vi "Tosca-Setup Devices.vi"(0 "Configuration file":path=path "C:/ProgramData/EPL/Tosca Defaults.ini", 2 "Parent VI":refnum<vi>, 7 "frame trigger?":bool) -> (6 "Changed":bool)   [LabVIEW 2020]
uses:
  TTL VIs/Typedefs/TTLControlledDevice XControl/TTLControlledDevice.xctl
  TTL VIs/Device Classes/Base Class/TTLControlledDevice.lvclass
  TTL VIs/Device Classes/WaterDelivery Class/TTLWaterDelivery.lvclass
  epl-vi-lib/Utility VIs/Controls/KTable/KTable.xctl
  TTL VIs/Device Classes/Base Class/TTLControlledDevice.lvclass/TTLControlledDevice.ctl
  epl-vi-lib/Connection VIs/Typedefs/CM-Endpoint.ctl
  e799b8b4-95e5-4a75-bcd5-f4c261b377d9.vi
  5e81ef1a-d4e7-4bbe-bc92-e5df060631d5.vi
  TTL VIs/Device Classes/Base Class/Read Name.vi
  TTL VIs/Device Classes/Base Class/Write Name.vi
  epl-vi-lib/Utility VIs/File IO VIs/Configuration File Wrapper VIs/Config-Read Key (string).vi
  epl-vi-lib/Utility VIs/File IO VIs/Configuration File Wrapper VIs/Config-Write Key (string).vi
  <vilib>/Comparison/Equal/Equal Functor/Equal Functor.lvclass
panel:
  in  "Add Button":bool
  in  "DO Port":u16(ring)=7 caption="Digital Output Port" items=["PXI1Slot3/port0"]
  in  "DI Port":u16(ring)=6 caption="Digital Input Port" items=["PXI1Slot3/port0", "PXI1Slot3/port1", "PXI1Slot3/port2"]
  in  "DO":u16(xcontrol)
  in  "DI":u16(xcontrol)
  in  "AO":u16(xcontrol)
  in  "AI":u16(xcontrol)
  in  "Apply Button":bool
  in  "Exit":bool
  in  "DigDevice 2":refnum<class "TTLControlledDevice.lvclass">(xcontrol)
  in  "DigDevice 1":refnum<class "TTLControlledDevice.lvclass">(xcontrol)=refnum
  in  "DigDevice 0":refnum<class "TTLControlledDevice.lvclass">(xcontrol)=refnum
  # "ANALOG"
  # "TTL-Controlled Devices"
  # "DIGITAL"
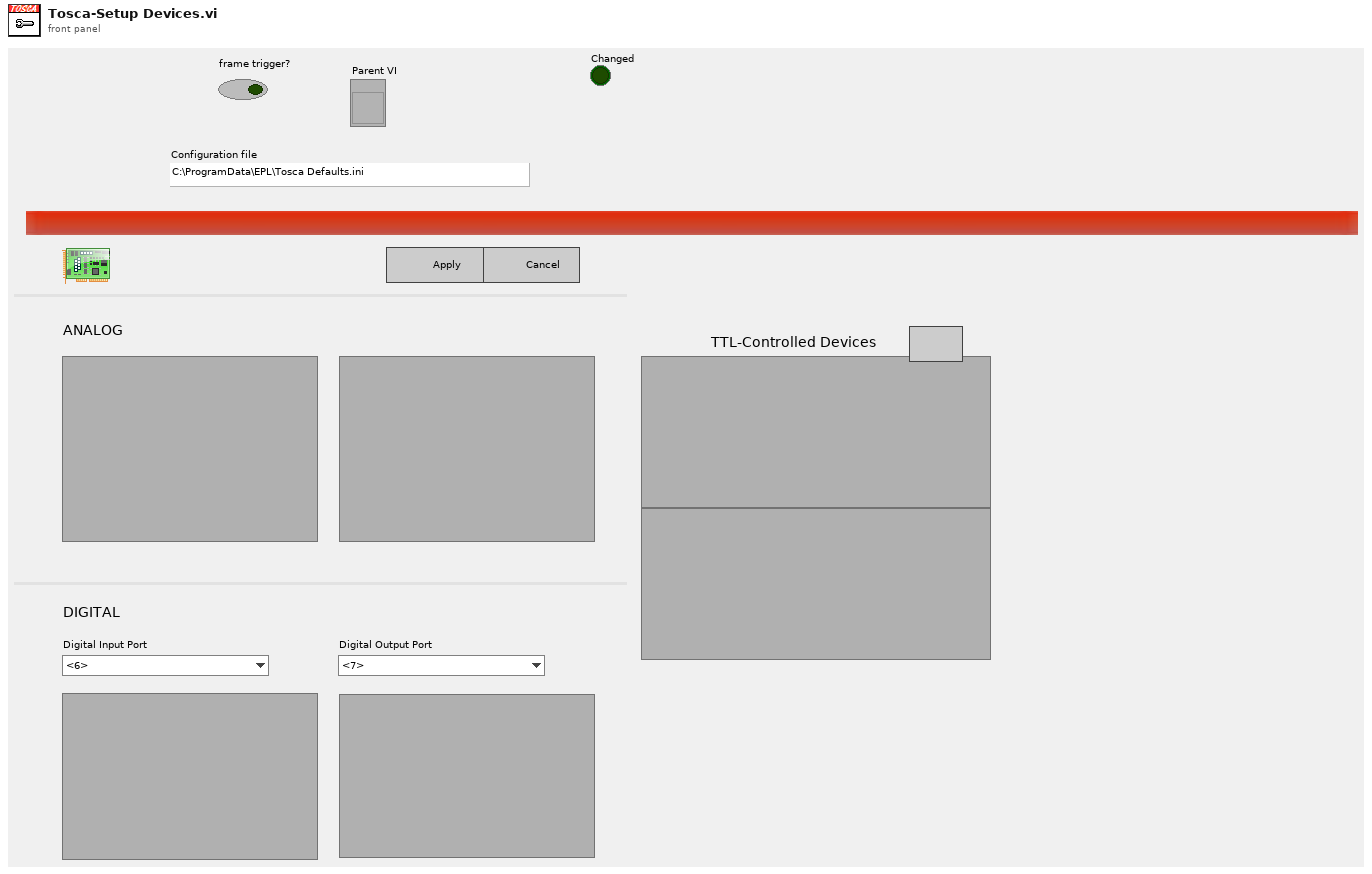
[diagram p1: front panel]
types:
  T1 = enum16{"Left Button", "Center Button", "Right Button", "Window Close"}
  T2 = typedef "CM-Endpoint.ctl" = cluster{"Name":string, "Device":string}
  T3 = enum8{"Enabled", "Disabled", "Disabled and Grayed Out"}
  T4 = typedef "CM-Connection.ctl" = cluster{"IOChannel":string, "Endpoint":string}
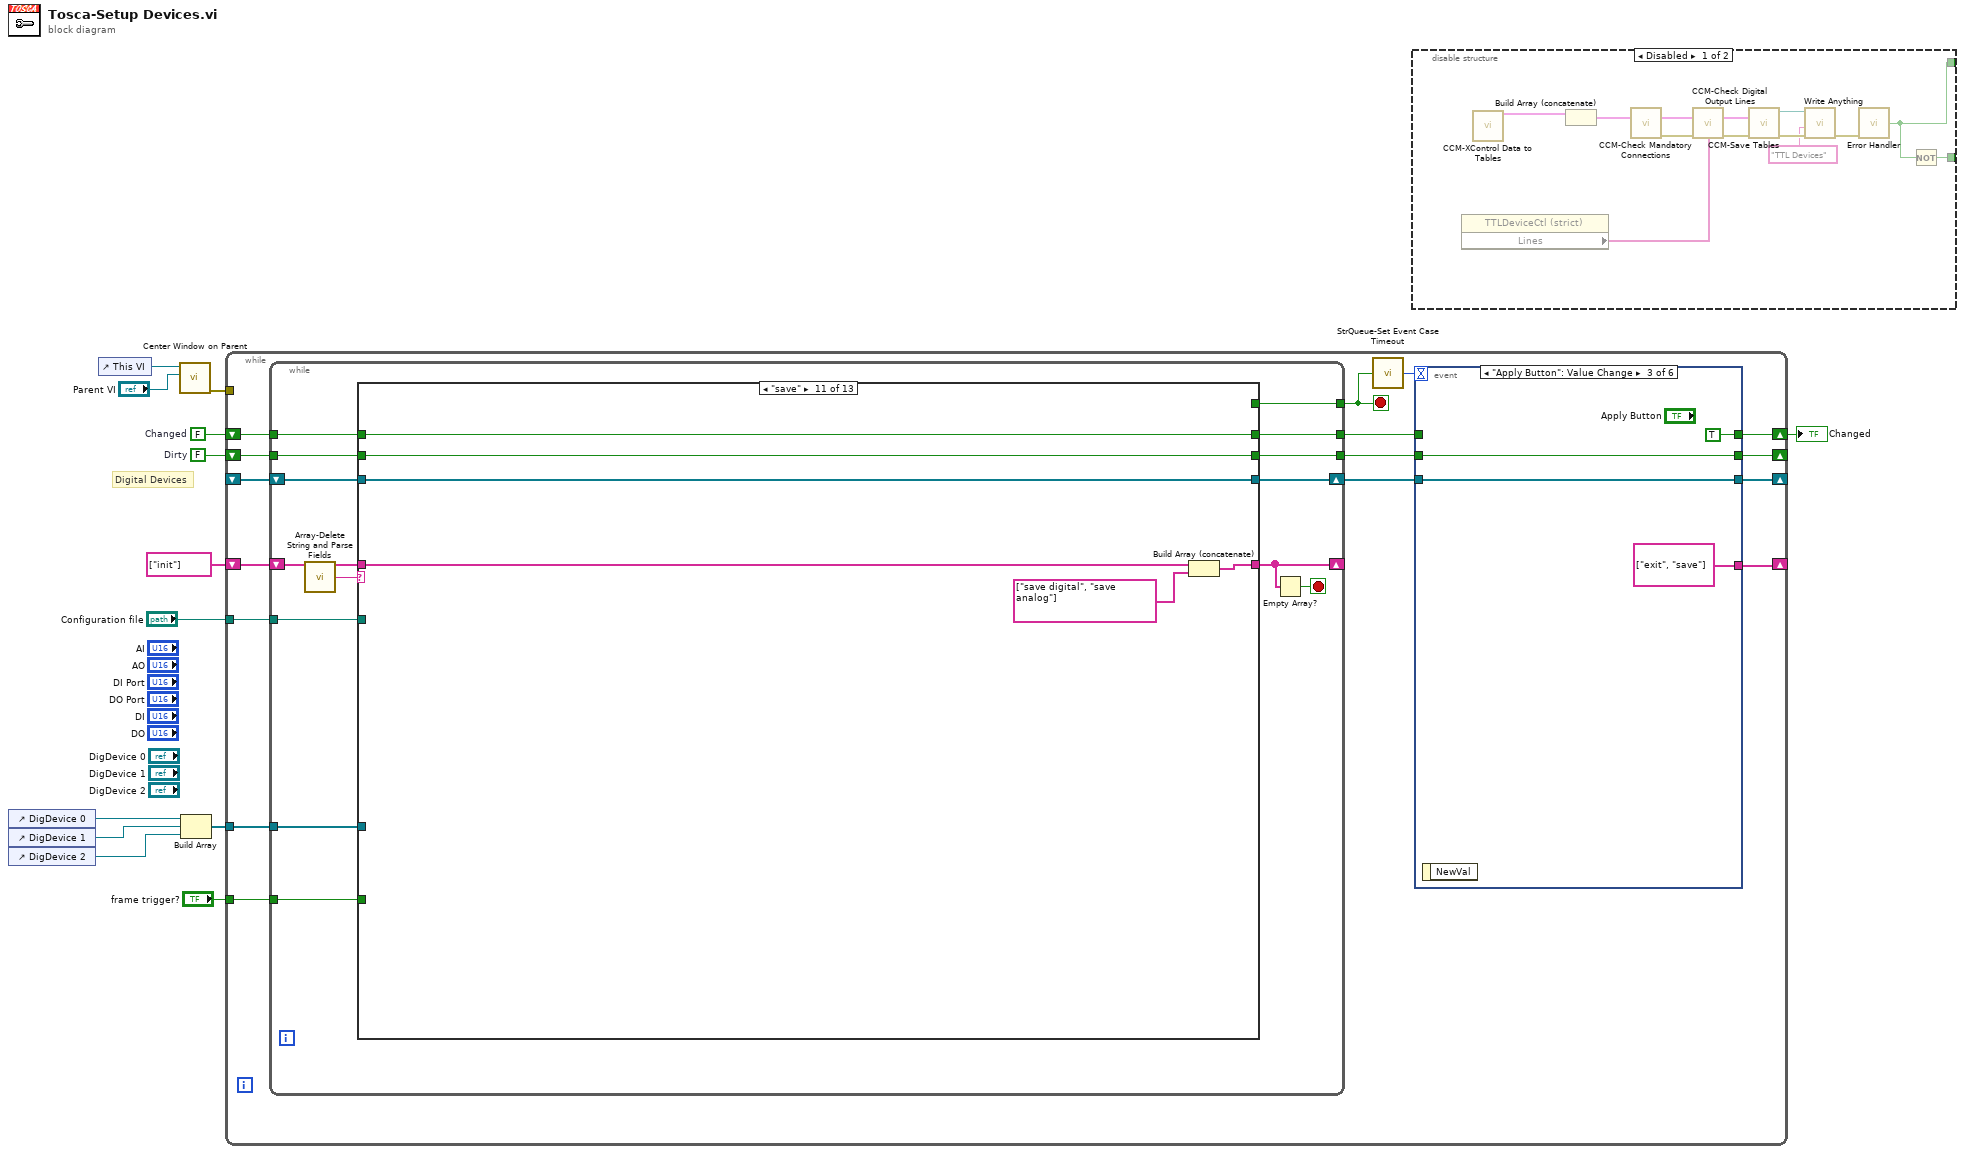
[diagram p0: block diagram]
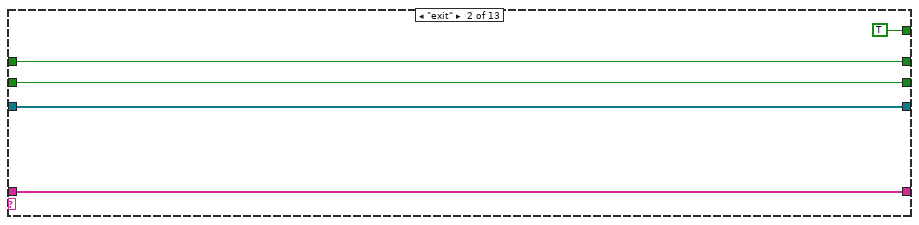
[diagram p3: hidden frame]
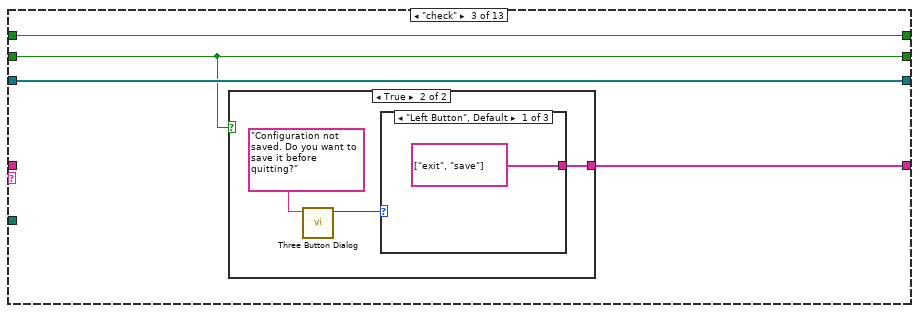
[diagram p4: hidden frame]
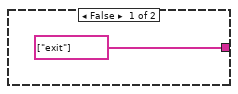
[diagram p5: hidden frame]
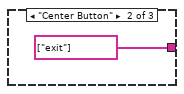
[diagram p6: hidden frame]
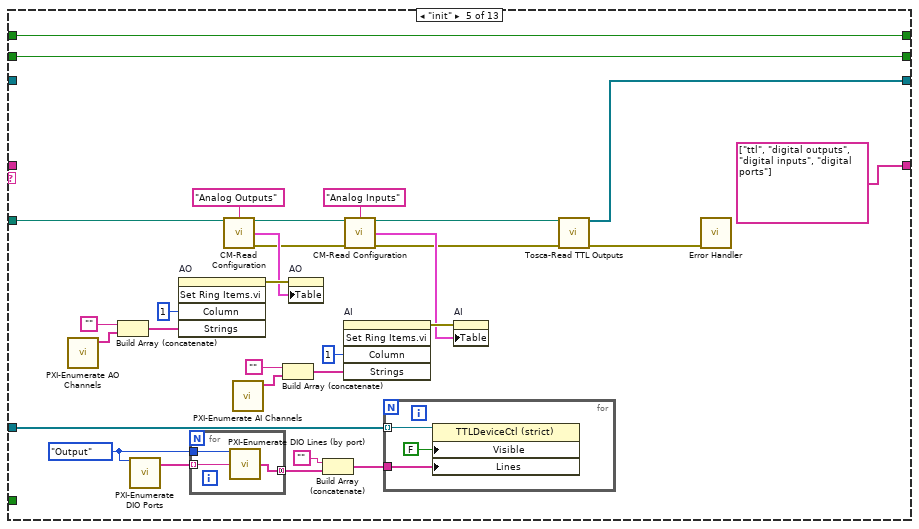
[diagram p9: hidden frame]
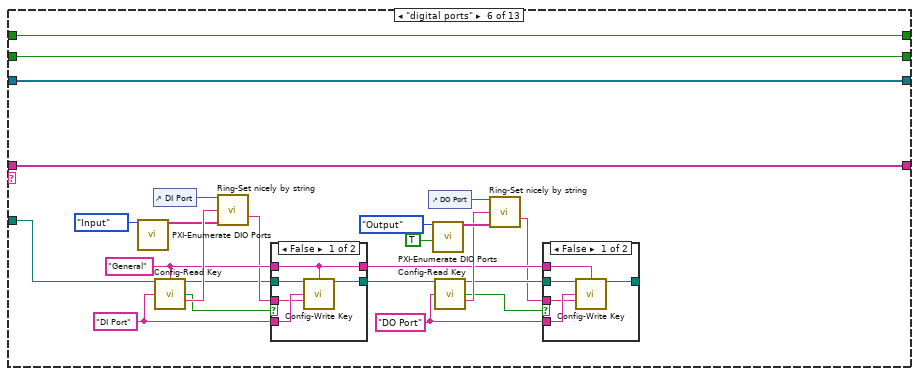
[diagram p10: hidden frame]
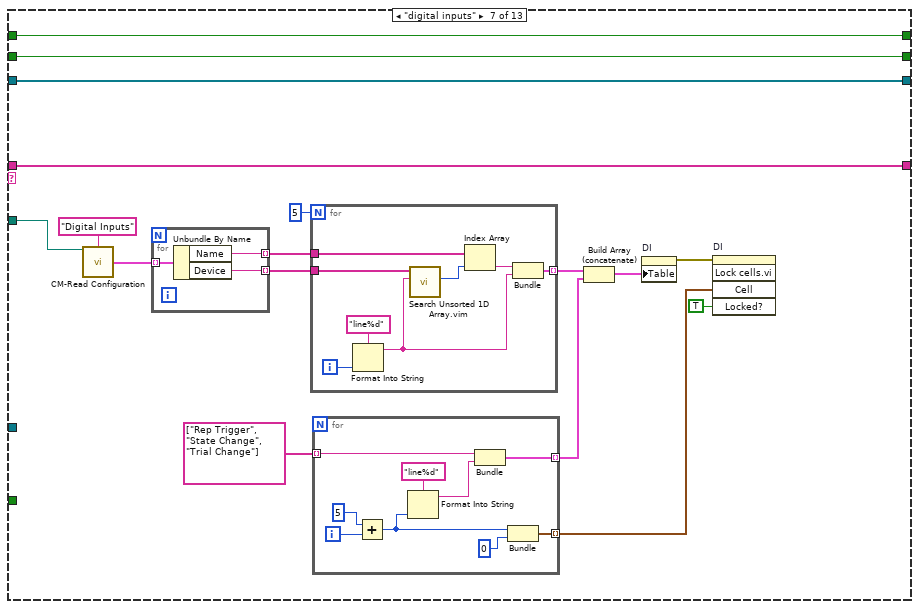
[diagram p13: hidden frame]
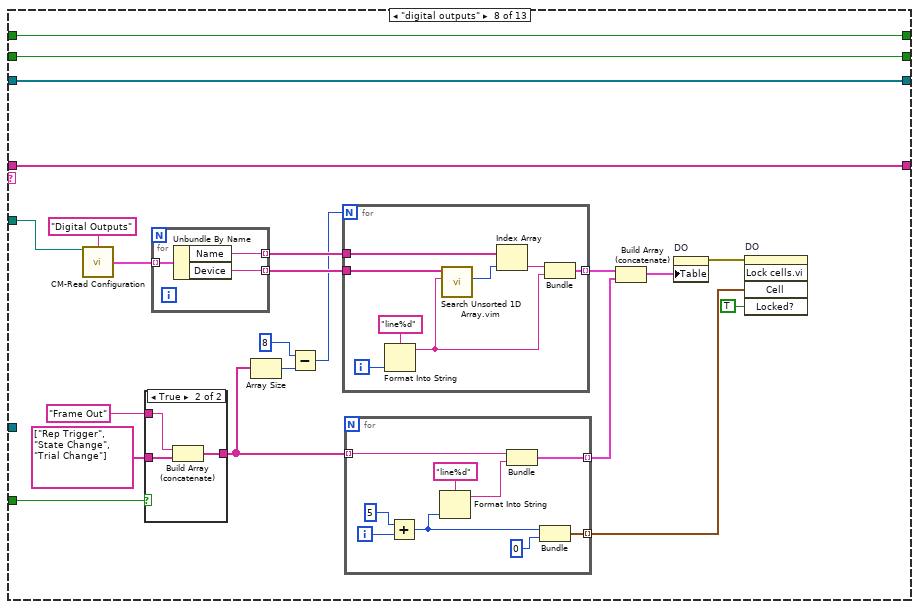
[diagram p14: hidden frame]
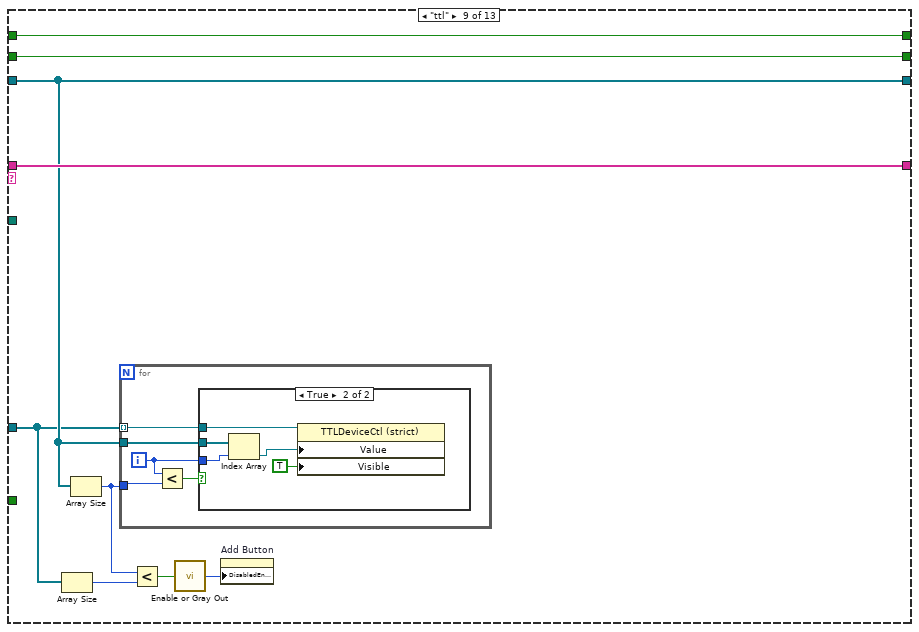
[diagram p16: hidden frame]
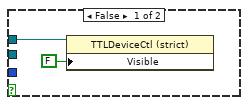
[diagram p17: hidden frame]
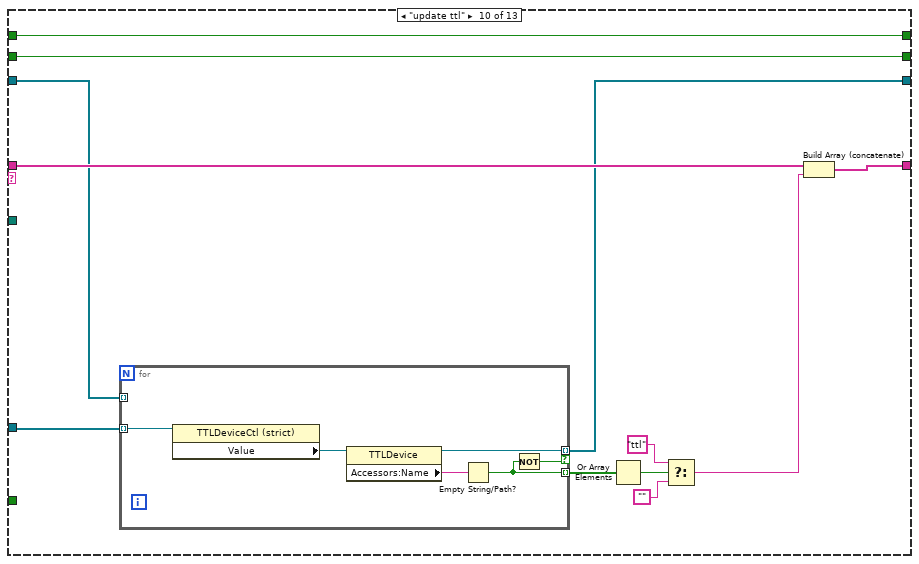
[diagram p18: hidden frame]
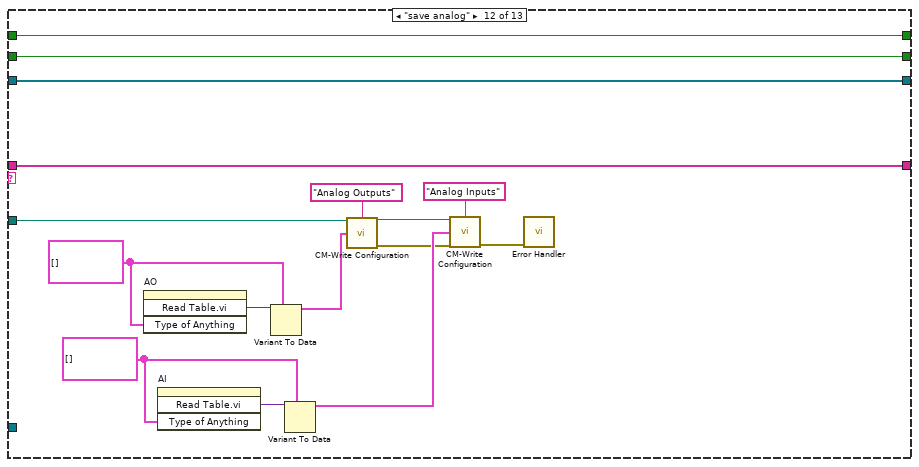
[diagram p19: hidden frame]
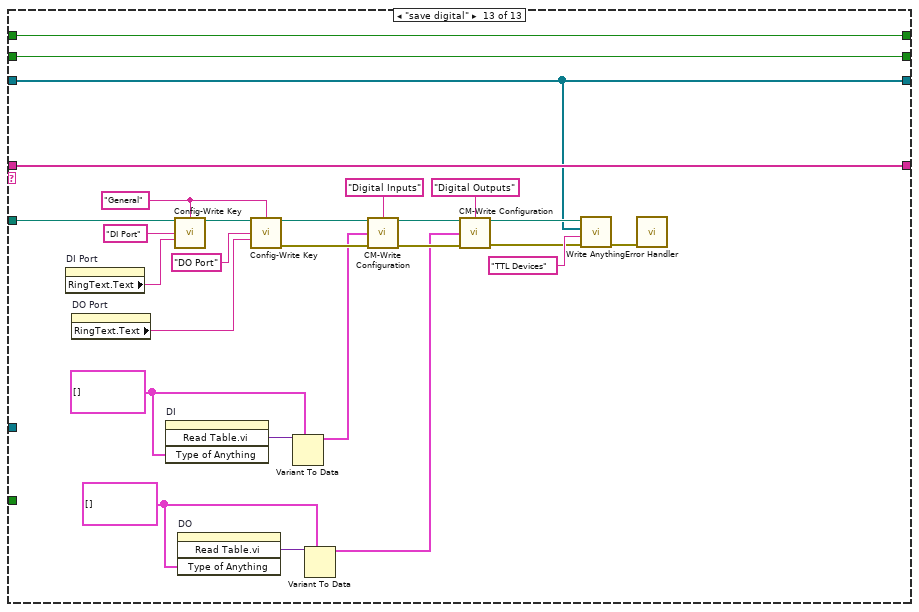
[diagram p20: hidden frame]
diagram:
  w11 = FALSE  # Changed
  w12 = FALSE  # Dirty
  # "Digital Devices"
  n1 = control-ref of="DigDevice 0"() -> (w9:refnum<vi>)
  n2 = control-ref of="DigDevice 1"() -> (w8:refnum<vi>)
  n3 = control-ref of="DigDevice 2"() -> (w7:refnum<vi>)
  n4 = control-ref of="This VI"() -> (w2:refnum<vi>)
  n5 = call "Center Window on Parent.vi"("Parent VI"="Parent VI", "VI in"=w2) -> ("error out"=w4:errorcluster)  [unwired: 8 in, 1 out]
  n6 = Build Array(w9, w8, w7) -> (w6:refnum<vi>[])
  n7 = while {
    shift-right: [w22] -> _
    shift-left: w12 -> [w27]
    tunnel: "Configuration file" -> [w16]
    shift-right: [w21] -> w10
    shift-left: w11 -> [w28]
    tunnel: w6 -> [w14]
    shift-right: [w23] -> _
    shift-left: _ -> [w26]
    shift-right: [w18] -> _
    shift-left: string[] ["init"] -> [w29]
    tunnel: w4 -> [_]
    tunnel: "frame trigger?" -> [w15]
    stop <- w24 stop-if-true
    n8 = while {
      shift-right: [w44] -> _
      shift-left: w29 -> [w41]
      tunnel: [w42] -> w24
      tunnel: w28 -> [w38]
      tunnel: w27 -> [w37]
      tunnel: [w35] -> w20
      tunnel: [w34] -> w19
      tunnel: w16 -> [w30]
      tunnel: w15 -> [w32]
      tunnel: w14 -> [w31]
      shift-right: [w33] -> w17
      shift-left: w26 -> [w36]
      stop <- w43 stop-if-true
      n9 = call "Array-Delete String and Parse Fields.vi"("Array in"=w41) -> ("Array out"=w40:string[], "Field 1"=w39:string)  [unwired: 10 in, 3 out]
      n10 = case shown="\"save\"" w39 {
        tunnel: w40 -> [w48 w53 _ w67 _ w105 w155 w197 w233 w257 w269 w285 w312]
        tunnel: [w48 w53 w54 w67 string[] ["ttl", "digital outputs", "digital inputs", "digital ports"] ("Array out") w105 w155 w197 w233 w251 w265 w285 w312] -> w44
        tunnel: [_ TRUE _ _ _ _ _ _ _ _ _ _ _] -> w42
        tunnel: w38 -> [w47 w51 w57 w66 w97 w128 w158 w200 w232 w256 w268 w284 w311]
        tunnel: w37 -> [w46 w50 w55 w65 w96 w127 w157 w199 w231 w255 w267 w283 w310]
        tunnel: w36 -> [w45 w49 w56 w64 _ w126 w156 w198 w230 w254 w266 w282 w289]
        tunnel: [w47 w51 w57 w66 w97 w128 w158 w200 w232 w256 w268 w284 w311] -> w35
        tunnel: [w46 w50 w55 w65 w96 w127 w157 w199 w231 w255 w267 w283 w310] -> w34
        tunnel: [w45 w49 w56 w64 w68 w126 w156 w198 w230 w252 w266 w282 w289] -> w33
        tunnel: w30 -> [_ _ _ _ w95 w104 w153 w195 _ _ _ w277 w307]
        tunnel: w32 -> [_ _ _ _ _ _ _ w184 _ _ _ _ _]
        tunnel: w31 -> [_ _ _ _ w72 _ _ _ w229 w253 _ _ _]
        frame "", Default {
        }
        frame "exit" {
        }
        frame "check" {
          n11 = case shown="True" w55 {
            tunnel: [string[] ["exit"] w59] -> w54
            frame False {
            }
            frame True {
              n12 = call <vilib>:"Three Button Dialog.vi"("message"="Configuration not saved. Do you want to save it before quitting?") -> ("Which Button?"=w60:T1)  [unwired: 10 in]
              n13 = case shown="\"Left Button\", Default" w60 {
                tunnel: [string[] ["exit", "save"] string[] ["exit"] _] -> w59
                frame "Left Button", Default {
                }
                frame "Center Button" {
                }
                frame "Right Button" {
                }
              }
            }
          }
        }
        frame "load" {
        }
        frame "init" {
          w75 = enum16{"Input", "Output"}."Output" ("Direction")
          n14 = call "PXI-Enumerate AO Channels.vi"() -> ("AO.PhysicalChans"=w92:tag[])  [unwired: 10 in, 1 out]
          n15 = Build Array (concatenate)("", w92) -> (w90:string[])
          n16 = call "PXI-Enumerate DIO Ports.vi"("Direction"=w75) -> ("Ports"=w74:tag[])  [unwired: 13 in, 1 out]
          n17 = invoke on="AO" class="KTable (strict)" method="Set Ring Items.vi"("Column"=1, "Strings"=w90) -> (error out=w94:errorcluster)  [unwired: 3 in, 4 out]
          n18 = for {
            tunnel: w74 -> [w99] mode=indexing
            tunnel: w75 -> [w100]
            tunnel: [w98] -> w76 mode=concatenating
            n19 = call "PXI-Enumerate DIO Lines (by port).vi"("Direction"=w100, "Port"=w99) -> ("Dev/Port/Lines"=w98:tag[])  [unwired: 11 in, 2 out]
          }
          n20 = call "CM-Read Configuration.vi"("Connection File Path"=w95, "Section"="Analog Outputs") -> ("Connection File Path thru"=w86:path, "Endpoints"=w89:T2[], "error out"=w85:errorcluster)  [unwired: 9 in, 2 out]
          n21 = call "PXI-Enumerate AI Channels.vi"() -> ("AI.PhysicalChans"=w82:tag[])  [unwired: 10 in, 1 out]
          n22 = Build Array (concatenate)("", w82) -> (w80:string[])
          n23 = property on="AO" class="KTable (strict)"(error in=w94, "Table"=w89) -> ()  [unwired: 1 in, 2 out]
          n24 = Build Array (concatenate)("", w76) -> (w77:string[])
          n25 = invoke on="AI" class="KTable (strict)" method="Set Ring Items.vi"("Column"=1, "Strings"=w80) -> (error out=w84:errorcluster)  [unwired: 3 in, 4 out]
          n26 = call "CM-Read Configuration.vi"("Connection File Path"=w86, "Section"="Analog Inputs", "error in (no error)"=w85) -> ("Connection File Path thru"=w71:path, "Endpoints"=w79:T2[], "error out"=w69:errorcluster)  [unwired: 8 in, 2 out]
          n27 = for {
            tunnel: w77 -> [w102]
            tunnel: w72 -> [w101] mode=indexing
            n28 = property class="TTLDeviceCtl (strict)"(reference=w101, "Visible"=FALSE, "Lines"=w102) -> ()  [unwired: 1 in, 2 out]
          }
          n29 = property on="AI" class="KTable (strict)"(error in=w84, "Table"=w79) -> ()  [unwired: 1 in, 2 out]
          n30 = call "Tosca-Read TTL Outputs.vi"("Connection File Path thru"=w71, "error in (no error)"=w69) -> ("Devices"=w68:refnum<class "TTLControlledDevice.lvclass">[], "error out"=w70:errorcluster)  [unwired: 12 in]
          n31 = call "Error Handler.vi"("error in (no error)"=w70) -> ()  [unwired: 12 in, 3 out]
        }
        frame "digital ports" {
          w110 = "DO Port" ("key")
          w116 = "DI Port" ("key")
          w117 = "General" ("section")
          n32 = call "PXI-Enumerate DIO Ports.vi"("Direction"=enum16{"Input", "Output"}."Input") -> ("Ports"=w121:tag[])  [unwired: 13 in, 1 out]
          n33 = control-ref of="DI Port"() -> (w107:refnum<vi>)
          n34 = call-poly "Config-Read Key.vi"("configuration file path"=w104, "section"=w117, "key"=w116) -> ("file path"=w114:path, "found?"=w118:bool, "value"=w122:string)  [unwired: 9 in, 1 out]
          n35 = call "Ring-Set nicely by string.vi"("Ring in"=w107, "Device"=w122, "Strings []"=w121) -> ("Selection"=w115:string)  [unwired: 8 in, 4 out]
          n36 = case shown="False" w118 {
            tunnel: w117 -> [w137 w141]
            tunnel: w116 -> [w139 _]
            tunnel: w115 -> [w138 _]
            tunnel: [w137 w141] -> w112
            tunnel: w114 -> [w136 w140]
            tunnel: [w135 w140] -> w113
            frame False {
              n37 = call-poly "Config-Write Key.vi"("configuration file path"=w136, "section"=w137, "key"=w139, "value"=w138) -> ("file path"=w135:path)  [unwired: 9 in, 2 out]
            }
            frame True {
            }
          }
          n38 = control-ref of="DO Port"() -> (w106:refnum<vi>)
          n39 = call "PXI-Enumerate DIO Ports.vi"("Direction"=enum16{"Input", "Output"}."Output", "Must be buffered"=TRUE) -> ("Ports"=w120:tag[])  [unwired: 12 in, 1 out]
          n40 = call-poly "Config-Read Key.vi"("configuration file path"=w113, "key"=w110) -> ("file path"=w111:path, "found?"=w108:bool, "value"=w119:string)  [unwired: 10 in, 1 out]
          n41 = call "Ring-Set nicely by string.vi"("Ring in"=w106, "Device"=w119, "Strings []"=w120) -> ("Selection"=w109:string)  [unwired: 8 in, 4 out]
          n42 = case shown="False" w108 {
            tunnel: w112 -> [w131 _]
            tunnel: w110 -> [w133 _]
            tunnel: w109 -> [w132 _]
            tunnel: w111 -> [w130 w134]
            tunnel: [w129 w134] -> _
            frame False {
              n43 = call-poly "Config-Write Key.vi"("configuration file path"=w130, "section"=w131, "key"=w133, "value"=w132) -> ("file path"=w129:path)  [unwired: 9 in, 2 out]
            }
            frame True {
            }
          }
        }
        frame "digital inputs" {
          n44 = call "CM-Read Configuration.vi"("Connection File Path"=w153, "Section"="Digital Inputs") -> ("Endpoints"=w152:T2[])  [unwired: 9 in, 4 out]
          n45 = for {
            tunnel: w152 -> [w178] mode=indexing
            tunnel: [w177] -> w150 mode=indexing
            tunnel: [w176] -> w149 mode=indexing
            n46 = Unbundle By Name(w178) -> ("Name"=w177:string, "Device"=w176:string)
          }
          n47 = for {
            N: 5 -> [_]
            tunnel: w150 -> [w172]
            tunnel: w149 -> [w173]
            tunnel: [w168] -> w147 mode=indexing
            i -> [w175]
            n48 = Format Into String(format string="line%d", w175) -> (resulting string=w169:string)  [unwired: 2 in, 1 out]
            n49 = call "Search Unsorted 1D Array.vim"("element"=w169, "unsorted 1D array"=w173) -> ("index of element"=w171:i32)  [unwired: 9 in]
            n50 = Index Array(array=w172, index=w171) -> (element=w170:string)
            n51 = Bundle("Name"=w170, w169) -> (w168:cluster{"Name":string, string})  [unwired: 1 in]
          }
          n52 = for {
            tunnel: string[] ["Rep Trigger", "State Change", "Trial Change"] -> [w163] mode=indexing
            tunnel: [w164] -> w146 mode=indexing
            tunnel: [w159] -> w143 mode=indexing
            i -> [w167]
            n53 = Add(x=5, y=w167) -> (x+y=w161:i32)
            n54 = Format Into String(format string="line%d", w161) -> (resulting string=w165:string)  [unwired: 2 in, 1 out]
            n55 = Bundle("String"=w163, w165) -> (w164:cluster{"String":string, string})  [unwired: 1 in]
            n56 = Bundle(w161, 0) -> (w159:cluster{i32, i32})  [unwired: 1 in]
          }
          n57 = Build Array (concatenate)(w147, w146) -> (w145:cluster{"String":string, string}[])
          n58 = property on="DI" class="KTable (strict)"("Table"=w145) -> (error out=w144:errorcluster)  [unwired: 2 in, 1 out]
          n59 = invoke on="DI" class="KTable (strict)" method="Lock cells.vi"(error in=w144, "Cell"=w143, "Locked?"=TRUE) -> ()  [unwired: 2 in, 5 out]
        }
        frame "digital outputs" {
          n60 = call "CM-Read Configuration.vi"("Connection File Path"=w195, "Section"="Digital Outputs") -> ("Endpoints"=w194:T2[])  [unwired: 9 in, 4 out]
          n61 = case shown="True" w184 {
            tunnel: string[] ["Rep Trigger", "State Change", "Trial Change"] -> [w201 w204]
            tunnel: [w201 w203] -> w181
            tunnel: "Frame Out" ("String") -> [_ w202]
            frame False {
            }
            frame True {
              n62 = Build Array (concatenate)(w202, w204) -> (w203:string[])
            }
          }
          n63 = for {
            tunnel: w194 -> [w224] mode=indexing
            tunnel: [w223] -> w193 mode=indexing
            tunnel: [w222] -> w192 mode=indexing
            n64 = Unbundle By Name(w224) -> ("Name"=w223:string, "Device"=w222:string)
          }
          n65 = Array Size(array=w181) -> (size(s)=w182:i32)
          n66 = Subtract(x=8, y=w182) -> (x-y=w179:i32)
          n67 = for {
            N: w179 -> [_]
            tunnel: w193 -> [w218]
            tunnel: w192 -> [w219]
            tunnel: [w214] -> w191 mode=indexing
            i -> [w221]
            n68 = Format Into String(format string="line%d", w221) -> (resulting string=w215:string)  [unwired: 2 in, 1 out]
            n69 = call "Search Unsorted 1D Array.vim"("element"=w215, "unsorted 1D array"=w219) -> ("index of element"=w217:i32)  [unwired: 9 in]
            n70 = Index Array(array=w218, index=w217) -> (element=w216:string)
            n71 = Bundle("Name"=w216, w215) -> (w214:cluster{"Name":string, string})  [unwired: 1 in]
          }
          n72 = for {
            tunnel: w181 -> [w209] mode=indexing
            tunnel: [w210] -> w190 mode=indexing
            tunnel: [w205] -> w187 mode=indexing
            i -> [w213]
            n73 = Add(x=5, y=w213) -> (x+y=w207:i32)
            n74 = Format Into String(format string="line%d", w207) -> (resulting string=w211:string)  [unwired: 2 in, 1 out]
            n75 = Bundle("String"=w209, w211) -> (w210:cluster{"String":string, string})  [unwired: 1 in]
            n76 = Bundle(w207, 0) -> (w205:cluster{i32, i32})  [unwired: 1 in]
          }
          n77 = Build Array (concatenate)(w191, w190) -> (w189:cluster{"String":string, string}[])
          n78 = property on="DO" class="KTable (strict)"("Table"=w189) -> (error out=w188:errorcluster)  [unwired: 2 in, 1 out]
          n79 = invoke on="DO" class="KTable (strict)" method="Lock cells.vi"(error in=w188, "Cell"=w187, "Locked?"=TRUE) -> ()  [unwired: 2 in, 5 out]
        }
        frame "ttl" {
          n80 = Array Size(array=w229) -> (size(s)=w227:i32)
          n81 = Array Size(array=w230) -> (size(s)=w228:i32)
          n82 = for {
            tunnel: w228 -> [w238]
            tunnel: w230 -> [w235]
            tunnel: w229 -> [w234] mode=indexing
            i -> [w236]
            n83 = Less?(x=w236, y=w238) -> (x < y?=w237:bool)
            n84 = case shown="True" w237 {
              tunnel: w236 -> [_ w245]
              tunnel: w235 -> [_ w243]
              tunnel: w234 -> [w239 w241]
              frame False {
                n85 = property class="TTLDeviceCtl (strict)"(reference=w239, "Visible"=FALSE) -> ()  [unwired: 1 in, 2 out]
              }
              frame True {
                n86 = Index Array(array=w243, index=w245) -> (element=w242:refnum<class "TTLControlledDevice.lvclass">)
                n87 = property class="TTLDeviceCtl (strict)"(reference=w241, "Value"=w242, "Visible"=TRUE) -> ()  [unwired: 1 in, 2 out]
              }
            }
          }
          n88 = Less?(x=w228, y=w227) -> (x < y?=w226:bool)
          n89 = call "Enable or Gray Out.vi"("Boolean"=w226) -> ("Disabled"=w225:T3)
          n90 = property on="Add Button" class="Bool"("DisabledEnum"=w225) -> ()  [unwired: 2 in, 2 out]
        }
        frame "update ttl" {
          n91 = for {
            tunnel: w254 -> [_] mode=indexing
            tunnel: w253 -> [w263] mode=indexing
            tunnel: [w260] -> w252 mode=indexing if=w259
            tunnel: [w258] -> w250 mode=indexing
            n92 = property class="TTLDeviceCtl (strict)"(reference=w263) -> ("Value"=w262:refnum<class "TTLControlledDevice.lvclass">)  [unwired: 1 in, 2 out]
            n93 = property class="TTLDevice"(reference=w262) -> (reference out=w260:refnum<class "TTLControlledDevice.lvclass">, "Accessors:Name"=w261:string)  [unwired: 1 in, 1 out]
            n94 = Empty String/Path?(string/path=w261) -> (empty?=w258:bool)
            n95 = Not(x=w258) -> (.not. x?=w259:bool)
          }
          n96 = Or Array Elements(Boolean array=w250) -> (logical OR=w249:bool)
          n97 = Select(t="ttl" ("String"), s=w249, f="") -> (s? t:f=w247:string)
          n98 = Build Array (concatenate)(w257, w247) -> (w251:string[])
        }
        frame "save" {
          n99 = Build Array (concatenate)(w269, string[] ["save digital", "save analog"]) -> (w265:string[])
        }
        frame "save analog" {
          w275 = T2[] [] ("Array")
          w280 = T2[] [] ("Array")
          n100 = invoke on="AO" class="KTable (strict)" method="Read Table.vi"("Type of Anything"=w280) -> ("Read Table.vi"=w281:variant)  [unwired: 3 in, 3 out]
          n101 = invoke on="AI" class="KTable (strict)" method="Read Table.vi"("Type of Anything"=w275) -> ("Read Table.vi"=w276:variant)  [unwired: 3 in, 3 out]
          n102 = Variant To Data(type=w280, Variant=w281) -> (data=w279:T2[])  [unwired: 1 in, 1 out]
          n103 = Variant To Data(type=w275, Variant=w276) -> (data=w274:T2[])  [unwired: 1 in, 1 out]
          n104 = call "CM-Write Configuration.vi"("Connection File Path"=w277, "Section"="Analog Outputs", "Endpoints"=w279) -> ("Path Out"=w271:path, "error out"=w272:errorcluster)  [unwired: 11 in]
          n105 = call "CM-Write Configuration.vi"("Connection File Path"=w271, "Section"="Analog Inputs", "Endpoints"=w274, "error in (no error)"=w272) -> ("error out"=w270:errorcluster)  [unwired: 10 in, 1 out]
          n106 = call "Error Handler.vi"("error in (no error)"=w270) -> ()  [unwired: 12 in, 3 out]
        }
        frame "save digital" {
          w292 = T2[] [] ("Array")
          w301 = T2[] [] ("Array")
          w309 = "General" ("section")
          n107 = property on="DI Port" class="Ring (strict)"() -> ("RingText.Text"=w306:string)  [unwired: 2 in, 2 out]
          n108 = property on="DO Port" class="Ring (strict)"() -> ("RingText.Text"=w303:string)  [unwired: 2 in, 2 out]
          n109 = invoke on="DI" class="KTable (strict)" method="Read Table.vi"("Type of Anything"=w301) -> ("Read Table.vi"=w302:variant)  [unwired: 3 in, 3 out]
          n110 = call-poly "Config-Write Key.vi"("configuration file path"=w307, "section"=w309, "key"="DI Port", "value"=w306) -> ("file path"=w305:path)  [unwired: 9 in, 2 out]
          n111 = invoke on="DO" class="KTable (strict)" method="Read Table.vi"("Type of Anything"=w292) -> ("Read Table.vi"=w293:variant)  [unwired: 3 in, 3 out]
          n112 = call-poly "Config-Write Key.vi"("configuration file path"=w305, "section"=w309, "key"="DO Port", "value"=w303) -> ("file path"=w299:path, "error out"=w298:errorcluster)  [unwired: 9 in, 1 out]
          n113 = Variant To Data(type=w301, Variant=w302) -> (data=w297:T2[])  [unwired: 1 in, 1 out]
          n114 = Variant To Data(type=w292, Variant=w293) -> (data=w291:T2[])  [unwired: 1 in, 1 out]
          n115 = call "CM-Write Configuration.vi"("Connection File Path"=w299, "Section"="Digital Inputs", "Endpoints"=w297, "error in (no error)"=w298) -> ("Path Out"=w295:path, "error out"=w294:errorcluster)  [unwired: 10 in]
          n116 = call "CM-Write Configuration.vi"("Connection File Path"=w295, "Section"="Digital Outputs", "Endpoints"=w291, "error in (no error)"=w294) -> ("Path Out"=w290:path, "error out"=w287:errorcluster)  [unwired: 10 in]
          n117 = call "Write Anything.vi"("Error In"=w287, "Section Name (Name of \"Anything\")"="TTL Devices" ("Section Name (Name of \"Anything\")"), "Anything"=w289, "Path (dialog)"=w290) -> ("Error Out"=w286:errorcluster)  [unwired: 6 in, 1 out]
          n118 = call "Error Handler.vi"("error in (no error)"=w286) -> ()  [unwired: 12 in, 3 out]
        }
      }
      n119 = Empty Array?(array=w44) -> (empty?=w43:bool)
    }
    n120 = call "StrQueue-Set Event Case Timeout.vi"("Quit"=w24) -> ("timeout"=w25:i32)  [unwired: 14 in]
    n121 = event shown="[2] \"Apply Button\": Value Change" {
      selector: _ -> [_ _ _ _ _ _]
      dyn-events: _ -> [_ _ _ _ _ _]
      timeout: w25 -> [_ _ _ _ _ _]
      tunnel: [w314 w320 w324 w326 TRUE ("Dirty") w343] -> w22
      tunnel: [w315 w319 TRUE w328 w331 w342] -> w21
      tunnel: [w313 w318 w323 w327 w330 w340] -> w23
      tunnel: w20 -> [w315 w319 _ w328 w331 w342]
      tunnel: w19 -> [w314 w320 w324 w326 _ w343]
      tunnel: [_ string[] ["check"] string[] ["exit", "save"] string[] ["check"] string[] ["update ttl"] string[] ["ttl"]] -> w18
      tunnel: w17 -> [w313 w318 w323 w327 w330 w337]
      event Timeout {
        n122 = event-data() -> ()  [unwired: 1 in, 1 out]
      }
      event Panel Close? {
        n123 = event-data() -> ()  [unwired: 1 in, 1 out]
        n124 = event-data("Discard?"=TRUE) -> ()  [unwired: 1 in, 1 out]
      }
      event "Apply Button": Value Change {
        n125 = event-data() -> ()  [unwired: 1 in, 1 out]
      }
      event "Exit": Value Change {
        n126 = event-data() -> ()  [unwired: 1 in, 1 out]
      }
      event "DigDevice 0", "DigDevice 1", "DigDevice 2": Value Change {
        n127 = event-data() -> ()  [unwired: 1 in, 1 out]
      }
      event "Add Button": Value Change {
        n128 = event-data() -> ()  [unwired: 1 in, 1 out]
        n129 = Array Size(array=w337) -> (size(s)=w336:i32)
        n130 = Increment(x=w336) -> (x+1=w335:i32)
        n131 = Format Into String(format string="TTL Device %d", w335) -> (resulting string=w333:string)  [unwired: 2 in, 1 out]
        n132 = property class="TTLDevice"(reference=refnum<class "TTLControlledDevice.lvclass"> refnum, "Accessors:Name"=w333) -> (reference out=w339:refnum<class "TTLControlledDevice.lvclass">)  [unwired: 1 in, 1 out]
        n133 = Build Array (concatenate)(w337, w339) -> (w340:refnum<class "TTLControlledDevice.lvclass">[])
      }
    }
  }
  "Changed" <- w10
  n134 = disable-structure shown="Disabled" {
    disable-tunnel: [w354 _] -> _
    disable-tunnel: [w353 _] -> _
    frame Disabled {
      n135 = property class="TTLDeviceCtl (strict)"() -> ("Lines"=w345:string[])  [unwired: 2 in, 2 out]
      n136 = call "CCM-XControl Data to Tables.vi"() -> ("Tables"=w356:cluster{"Table":T4[]}[])  [unwired: 15 in]
      n137 = Build Array (concatenate)(w356) -> (w355:cluster{"Table":T4[]}[])  [unwired: 1 in]
      n138 = call "CCM-Check Mandatory Connections.vi"("Tables"=w355) -> ("Tables thru"=w346:cluster{"Table":T4[]}[], "error out"=w348:errorcluster)  [unwired: 13 in]
      n139 = call "CCM-Check Digital Output Lines.vi"("Tables"=w346, "error in (no error)"=w348, "DO Lines"=w345) -> ("Tables thru"=w344:cluster{"Table":T4[]}[], "error out"=w347:errorcluster)  [unwired: 11 in]
      n140 = call "CCM-Save Tables.vi"("Tables"=w344, "error in (no error)"=w347) -> ("file path"=w350:path, "error out"=w351:errorcluster)  [unwired: 12 in]
      n141 = call "Write Anything.vi"("Error In"=w351, "Section Name (Name of \"Anything\")"="TTL Devices" ("Section Name (Name of \"Anything\")"), "Path (dialog)"=w350) -> ("Error Out"=w352:errorcluster)  [unwired: 7 in, 1 out]
      n142 = call "Error Handler.vi"("error in (no error)"=w352) -> ("error?"=w354:bool)  [unwired: 12 in, 2 out]
      n143 = Not(x=w354) -> (.not. x?=w353:bool)
    }
    frame Enabled {
    }
  }
